vi "Ogrod_zmienne.vi"() -> ()   [LabVIEW 2023]
panel:
  in  "Czas podlewania":dbl
  in  "Czas podlewania reczny":dbl
  in  "Ustaw":bool
  in  "Sekcja tryb reczny":dbl
  in  "Podlewaj tryb reczny":bool
  in  "Podlewaj":bool
  in  "Liczba sekcji":dbl
  in  "Minuta":dbl
  in  "Godzina":dbl
  in  "Rok":dbl
  in  "Miesiac":dbl
  in  "Dzien":dbl
  in  "Czas podlewania":dbl
  in  "Powierzchnia":dbl
  in  "Ilosc zraszaczy":dbl
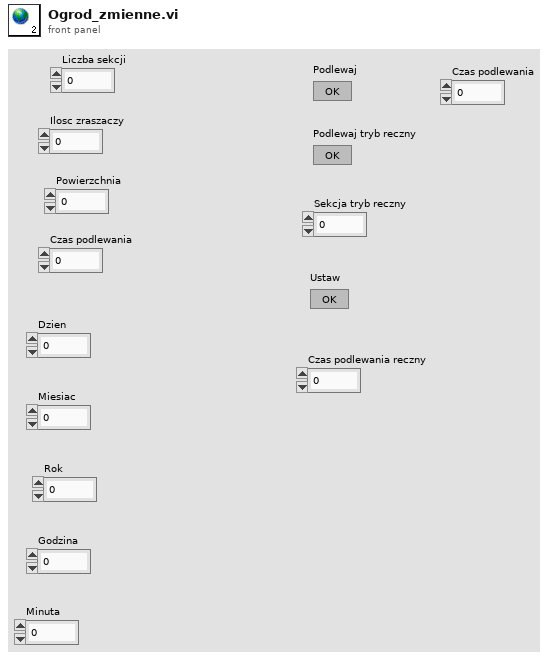
[diagram p1: front panel]
diagram:
